vi "dense-top.vi"(11 "x_dense":T1) -> (3 "y_out":T1)   [LabVIEW 2020]
uses:
  <vilib>/Analysis/Matrix/Datatypes/RealMatrix.ctl
  <vilib>/Analysis/Matrix/Numeric/Conversions/Array To Matrix - RA2.vi
  <vilib>/Analysis/Matrix/Numeric/Multiply/Multiply - RM,RM.vi
  <vilib>/Analysis/Matrix/Numeric/Multiply/Multiply - R,RM.vi
  <vilib>/Analysis/Matrix/NI_Matrix.lvlib
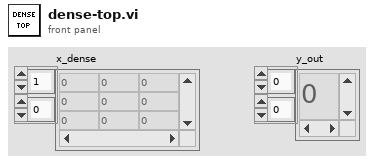
[diagram p1: front panel]
types:
  T1 = typedef "NI_Matrix.lvlib/RealMatrix.ctl" = dbl[][]
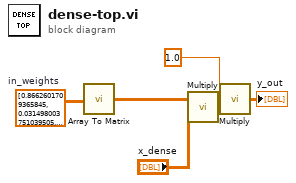
[diagram p0: block diagram]
diagram:
  w2 = dbl[][] [[0.8662601709365845, 0.031498003751039505, -0.6739006638526917, 0.13976523280143738, -0.4540349245071411, -0.33356979489326477, -0.9548949003219604, -0.4968436360359192, 0.5050259828567505, 0.393038809299469, 0.12224956601858139, -0.5444044470787048, -0.02216361276805401, 0.035558123141527176, -0.8653411865234375]]  # in_weights
  n1 = call-poly <vilib>:"Array To Matrix.vi"("Real 2D Array"=w2) -> ("Real Matrix"=w1:T1)
  n2 = call-poly <vilib>:"Multiply.vi"("Real Matrix B"="x_dense", "Real Matrix A"=w1) -> ("A * B"=w5:T1)
  n3 = call-poly <vilib>:"Multiply.vi"("Real Matrix A"=w5, "Real Scalar c"=1.0) -> ("c * A"=→"y_out":T1)
